vi "example test.vi"() -> ()   [LabVIEW 2013, in "Scan Engine tests.lvlib"]
uses:
  Scan Engine tests.lvlib
  configuration/Scan Engine configuration.lvclass
  <vilib>/NI/Tag Bus Module Framework/channel/channel classification.ctl
  <vilib>/NI/Tag Bus/tag/Data Type.ctl
  execution/Scan Engine runtime.lvclass
  configuration/Line.ctl
  <vilib>/NI/Tag Bus Module Framework/channel/TBM channel.lvclass
  <vilib>/NI/Tag Bus/dictionary/data dictionary.lvclass/data dictionary.ctl
  <vilib>/NI/Tag Bus/dictionary/lookup polymorphs/locate double.vi
  <vilib>/NI/Tag Bus/table/data polymorphs/write one/write Double.vi
  <vilib>/NI/Tag Bus/table/data polymorphs/read one/read Double.vi
  <vilib>/NI/Tag Bus/dictionary/search/find data index.vi
  <vilib>/NI/Tag Bus/dictionary/search/search string list.vi
  <vilib>/NI/Tag Bus/dictionary/tag not found.vi
  <vilib>/NI/Tag Bus/tag/tag descriptor.lvclass
  <vilib>/NI/Tag Bus/dictionary/data dictionary.lvclass
  <vilib>/NI/Tag Bus/table/data table.lvlib
  <vilib>/NI/Configuration Framework/serializable configuration/NISE_CEF_serializable configuration.lvclass
panel:
  out "final error":errorcluster
  out "output error":errorcluster
  out "input error":errorcluster
  out "output lookup error":errorcluster
  out "no data written":bool
  out "input lookup error":errorcluster
  out "init error":errorcluster
  out "correct execution settings":bool
  out "serialization problem":errorcluster
  out "invalid configuration":errorcluster
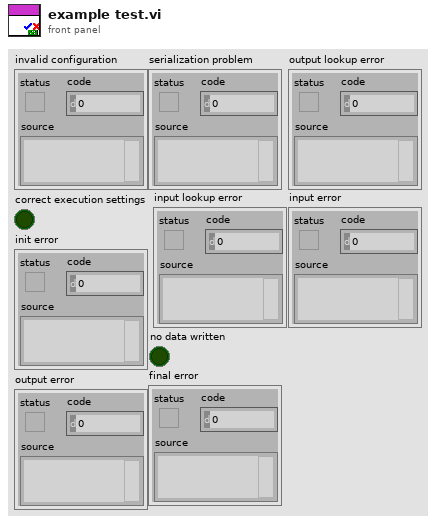
[diagram p1: front panel]
types:
  T1 = typedef "Scan Engine configuration.lvclass/Line.ctl" = cluster{"channel":refnum<class "TBM channel.lvclass">, "Tag":string}
  T2 = typedef "TBM channel.lvclass/channel classification.ctl" = enum16{"input data", "output data", "processing parameter", "processing result"}
  T3 = typedef "tag bus.lvlib/tag descriptor.lvclass/Data Type.ctl" = enum16{"Double", "Single", "I64", "I32", "I16", "I8", "U64", "U32", "U16", "U8", "Boolean", "String", "Array of Double", "Array of Single", "Array of I64", "Array of I32", "Array of I16", "Array of I8", "Array of U64", "Array of U32", "Array of U16", "Array of U8", "Array of Boolean", "Array of String"}
  T4 = typedef "TBM channel.lvclass/data tables.ctl" = cluster{"input data":T5, "processing parameter":T5, "processing result":T5, "output data":T5}
  T5 = typedef "tag bus.lvlib/dictionary table pair.ctl" = cluster{"data dictionary":refnum<class "data dictionary.lvclass">, "data table":T6}
  T6 = typedef "tag bus.lvlib/data table.lvlib/data table.ctl" = cluster{"Double":dbl[], "Single":sgl[], "I64":i64[], "I32":i32[], "I16":i16[], "I8":i8[], "U64":u64[], "U32":u32[], "U16":u16[], "U8":u8[], "Boolean":bool[], "String":string[], "Array of Double":cluster{"DBL Array":dbl[]}[], "Array of Single":cluster{"SGL Array":sgl[]}[], "Array of I64":cluster{"I64 Array":i64[]}[], "Array of I32":cluster{"I32 Array":i32[]}[], "Array of I16":cluster{"I16 Array":i16[]}[], "Array of I8":cluster{"I8 Array":i8[]}[], "Array of U64":cluster{"U64 Array":u64[]}[], "Array of U32":cluster{"U32 Array":u32[]}[], "Array of U16":cluster{"U16 Array":u16[]}[], "Array of U8":cluster{"U8 Array":u8[]}[], "Array of Boolean":cluster{"Boolean Array":bool[]}[], "Array of String":cluster{"String Array":string[]}[]}
  T7 = typedef "TBM module execution interface.lvclass/execution settings.ctl" = cluster{"reads inputs":bool, "processes data":bool, "writes outputs":bool}
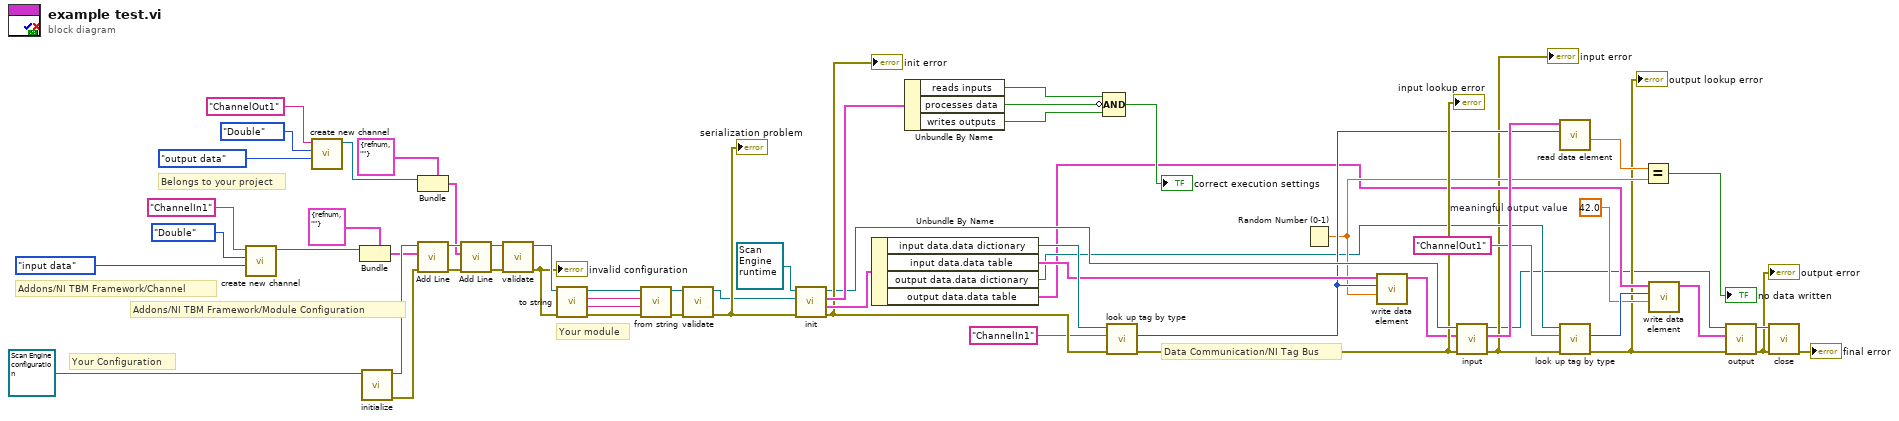
[diagram p0: block diagram]
diagram:
  w20 = 42.0  # meaningful output value
  # "Data Communication/NI Tag Bus"
  # "Your module"
  # "Your Configuration"
  # "Addons/NI TBM Framework/Module Configuration"
  # "Belongs to your project"
  # "Addons/NI TBM Framework/Channel"
  n1 = call <vilib>:"create new channel.vi"("channel classification"=channel_classification."input data", "data type"=Data_Type."Double", "channel name"="ChannelIn1") -> ("channel"=w6:refnum<class "TBM channel.lvclass">)  [unwired: 8 in]
  n2 = call <vilib>:"create new channel.vi"("channel classification"=channel_classification."output data", "data type"=Data_Type."Double", "channel name"="ChannelOut1") -> ("channel"=w4:refnum<class "TBM channel.lvclass">)  [unwired: 8 in]
  n3 = Bundle(cluster=T1 {"channel"=refnum, "Tag"=""} ("Line"), "channel"=w6) -> (w5:T1)  [unwired: 1 in]
  n4 = call <vilib>:"initialize.vi"("configuration in"=refnum<class "Scan Engine configuration.lvclass"> refnum ("tag bus configurable plugin module configuration")) -> ("error out"=w8:errorcluster, "configuration out"=w9:refnum<class "Scan Engine configuration.lvclass">)  [unwired: 8 in, 1 out]
  n5 = Bundle(cluster=T1 {"channel"=refnum, "Tag"=""} ("Line"), "channel"=w4) -> (w3:T1)  [unwired: 1 in]
  n6 = call "Add Line.vi"("error in"=w8, "Line"=w5, "Scan Engine configuration in"=w9) -> ("error out"=w10:errorcluster, "Scan Engine configuration out"=w12:refnum<class "Scan Engine configuration.lvclass">)  [unwired: 7 in]
  n7 = call "Add Line.vi"("error in"=w10, "Line"=w3, "Scan Engine configuration in"=w12) -> ("error out"=w7:errorcluster, "Scan Engine configuration out"=w11:refnum<class "Scan Engine configuration.lvclass">)  [unwired: 7 in]
  n8 = call-dynamic "validate.vi"("error in"=w7, "Scan Engine configuration in"=w11) -> ("error out"=w53:errorcluster, "Scan Engine configuration out"=w54:refnum<class "Scan Engine configuration.lvclass">)  [unwired: 8 in]
  "invalid configuration" <- w53
  n9 = call-dynamic "to string.vi"("error in"=w53, "Scan Engine configuration in"=w54) -> ("error out"=w49:errorcluster, "data"=w50:string, "version"=w51:string, "Scan Engine configuration out"=w52:refnum<class "Scan Engine configuration.lvclass">)  [unwired: 6 in]
  n10 = call-dynamic "from string.vi"("error in"=w49, "data"=w50, "version"=w51, "Scan Engine configuration in"=w52) -> ("error out"=w47:errorcluster, "Scan Engine configuration out"=w48:refnum<class "Scan Engine configuration.lvclass">)  [unwired: 6 in]
  n11 = call-dynamic "validate.vi"("error in"=w47, "Scan Engine configuration in"=w48) -> ("error out"=w45:errorcluster, "Scan Engine configuration out"=w44:refnum<class "Scan Engine configuration.lvclass">)  [unwired: 8 in]
  "serialization problem" <- w45
  n12 = call-dynamic "init.vi"("error in"=w45, "TBM module configuration in"=w44, "Scan Engine runtime in"=refnum<class "Scan Engine runtime.lvclass"> refnum ("tag bus configurable plugin module")) -> ("error out"=w36:errorcluster, "data allocations"=w38:T4, "execution settings"=w43:T7, "Scan Engine runtime out"=w33:refnum<class "Scan Engine runtime.lvclass">)  [unwired: 5 in]
  "init error" <- w36
  n13 = Unbundle By Name(w38) -> ("input data.data dictionary"=w37:refnum<class "data dictionary.lvclass">, "input data.data table"=w34:T6, "output data.data dictionary"=w25:refnum<class "data dictionary.lvclass">, "output data.data table"=w22:T6)
  n14 = Unbundle By Name(w43) -> ("reads inputs"=w40:bool, "processes data"=w42:bool, "writes outputs"=w41:bool)
  n15 = Compound Arithmetic op=AND(w40, invert w42, w41) -> (→"correct execution settings":bool)
  n16 = call-poly <vilib>:"look up tag by type.vi"("error in"=w36, "name"="ChannelIn1" ("channel name"), "data dictionary in"=w37) -> ("error out"=w32:errorcluster, "index"=w29:i32)  [unwired: 6 in, 1 out]
  "input lookup error" <- w32
  n17 = Random Number (0-1)() -> (number: 0 to 1=w28:dbl)
  n18 = call-poly <vilib>:"write data element.vi"("value"=w28, "index"=w29, "data table in"=w34) -> ("data table out"=w31:T6)  [unwired: 8 in]
  n19 = call-dynamic "input.vi"("error in"=w32, "data table in"=w31, "Scan Engine runtime in"=w33) -> ("error out"=w21:errorcluster, "data table out"=w30:T6, "Scan Engine runtime out"=w18:refnum<class "Scan Engine runtime.lvclass">)  [unwired: 6 in]
  "input error" <- w21
  n20 = call-poly <vilib>:"read data element.vi"("index"=w29, "data table in"=w30) -> ("value"=w27:dbl)  [unwired: 8 in, 1 out]
  n21 = call-poly <vilib>:"look up tag by type.vi"("error in"=w21, "name"="ChannelOut1" ("channel name"), "data dictionary in"=w25) -> ("error out"=w19:errorcluster, "index"=w23:i32)  [unwired: 6 in, 1 out]
  "output lookup error" <- w19
  n22 = Equal?(x=w27, y=w28) -> (x = y?=→"no data written":bool)
  n23 = call-poly <vilib>:"write data element.vi"("value"=w20, "index"=w23, "data table in"=w22) -> ("data table out"=w17:T6)  [unwired: 8 in]
  n24 = call-dynamic "output.vi"("error in"=w19, "data table in"=w17, "Scan Engine runtime in"=w18) -> ("error out"=w15:errorcluster, "Scan Engine runtime out"=w16:refnum<class "Scan Engine runtime.lvclass">)  [unwired: 6 in, 1 out]
  "output error" <- w15
  n25 = call-dynamic "close.vi"("error in"=w15, "Scan Engine runtime in"=w16) -> ("error out"=→"final error":errorcluster)  [unwired: 9 in]
